vi "SetMotor.vi"(8 "tics":u8, 9 "direction":u8, 10 "pwm":u8, 11 "port":enum8{"M1", "M2", "M3", "M4", "M5", "M6"}(ring)) -> (3 "set motor packet":string)   [LabVIEW 2018]
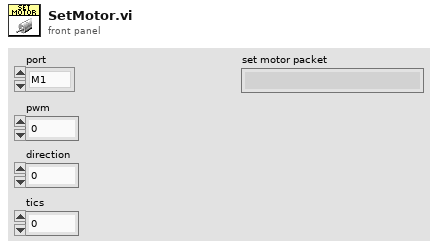
[diagram p1: front panel]
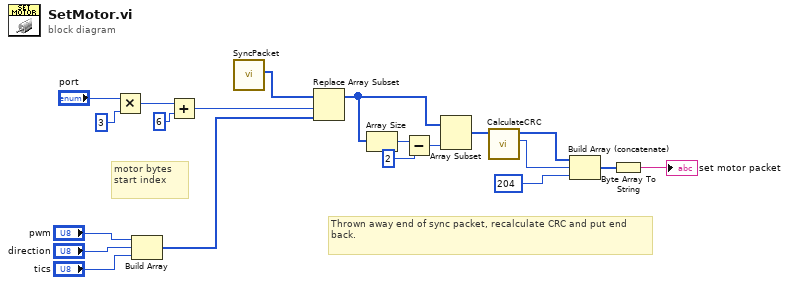
[diagram p0: block diagram]
diagram:
  # "Thrown away end of sync packet, recalculate CRC and put end back."
  # "motor bytes start index"
  n1 = Multiply(x="port", y=u8 3) -> (x*y=w19:u8)
  n2 = Build Array("pwm", "direction", "tics") -> (w12:u8[])
  n3 = Add(x=w19, y=u8 6) -> (x+y=w17:u8)
  n4 = call "SyncPacket.vi"() -> ("sync packet array"=w16:u8[])  [unwired: 10 in, 1 out]
  n5 = Replace Array Subset(array=w16, new element=w12, index=w17) -> (w10:u8[])
  n6 = Array Size(array=w10) -> (size(s)=w9:i32)
  n7 = Subtract(x=w9, y=2) -> (x-y=w7:i32)
  n8 = Array Subset(array=w10, length=w7) -> (w6:u8[])  [unwired: 1 in]
  n9 = call "CalculateCRC.vi"("data in"=w6) -> ("CRC"=w3:u8, "data out"=w4:u8[])  [unwired: 9 in]
  n10 = Build Array (concatenate)(w4, w3, u8 204) -> (w2:u8[])
  n11 = Byte Array To String(unsigned byte array=w2) -> (string=→"set motor packet":string)
